vi "Instrument Type ID.vi"() -> (1 "instrument type id":string="niDigitalPattern")   [LabVIEW 2020, in "NI Session Management niDigital.lvlib"]
uses:
  NI Session Management niDigital.lvlib
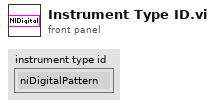
[diagram p1: front panel]
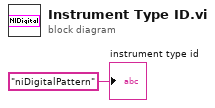
[diagram p0: block diagram]
diagram:
  "instrument type id" <- "niDigitalPattern" ("instrument type id")
